vi "BSA_Setup_Options.vi"() -> (0 "IP Addresses":string[](array[string]), 1 "Channel Numbers":i32[](array[numeric]), 2 "Full BSA Strings":string[](array[string]), 3 "BSA Types":string[](array[string]), 4 "Record Length":dbl[](array[numeric])=[16.0, 32.0, 64.0, 128.0, 256.0, 512.0, 1024.0])   [LabVIEW 2022 SP3]
uses:
  <vilib>/Utility/error.llb/Trim Whitespace One-Sided.vi
  Globals/Constants_global.vi
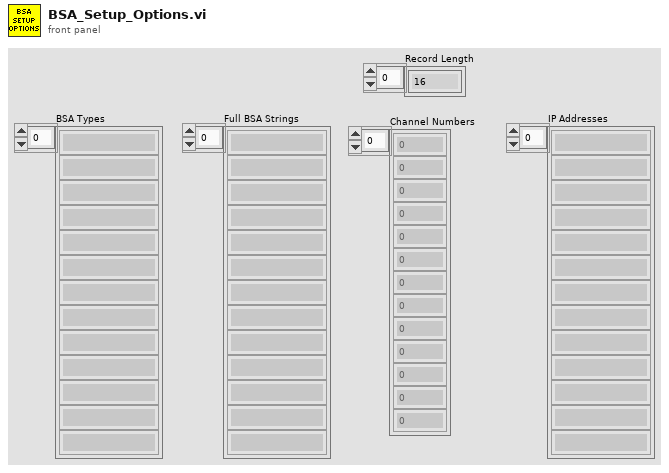
[diagram p1: front panel]
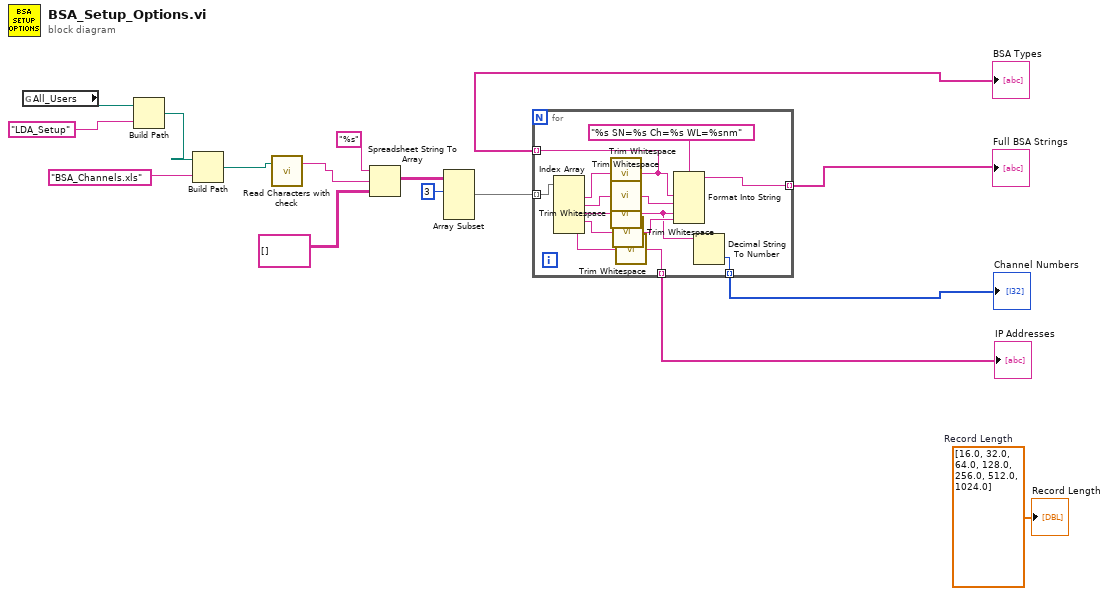
[diagram p0: block diagram]
diagram:
  w12 = dbl[] [16.0, 32.0, 64.0, 128.0, 256.0, 512.0, 1024.0]  # Record Length
  n1 = global read "Constants_global.vi" "All_Users"() -> (w11:path)
  n2 = Build Path(base path=w11, name or relative path="LDA_Setup") -> (appended path=w10:path)
  n3 = Build Path(base path=w10, name or relative path="BSA_Channels.xls") -> (appended path=w2:path)
  n4 = call "Read Characters with check.vi"("file (use dialog)"=w2) -> ("Read String"=w1:string)  [unwired: 1 in, 1 out]
  n5 = Spreadsheet String To Array(format string="%s", spreadsheet string=w1, array type (2D Dbl)=string[][] []) -> (array=w6:string[][])  [unwired: 1 in]
  n6 = Array Subset(array=w6, index (row)=3 ("index")) -> (w8:string[][])  [unwired: 3 in]
  n7 = for {
    tunnel: w8 -> [w30] mode=indexing
    tunnel: [w28] -> w16 mode=indexing
    tunnel: [w19] -> w14 mode=indexing
    tunnel: [w21] -> w15 mode=indexing
    tunnel: [w17] -> w13 mode=indexing
    n8 = Index Array(array=w30) -> (element #1=w22:string, element #2=w27:string, element #3=w25:string, element #4=w24:string, element #5=w20:string)  [unwired: 5 in]
    n9 = call <vilib>:"Trim Whitespace.vi"("string"=w22) -> ("trimmed string"=w21:string)  [unwired: 1 in]
    n10 = call <vilib>:"Trim Whitespace.vi"("string"=w27) -> ("trimmed string"=w26:string)  [unwired: 1 in]
    n11 = call <vilib>:"Trim Whitespace.vi"("string"=w25) -> ("trimmed string"=w18:string)  [unwired: 1 in]
    n12 = call <vilib>:"Trim Whitespace.vi"("string"=w24) -> ("trimmed string"=w23:string)  [unwired: 1 in]
    n13 = call <vilib>:"Trim Whitespace.vi"("string"=w20) -> ("trimmed string"=w19:string)  [unwired: 1 in]
    n14 = Format Into String(format string="%s SN=%s Ch=%s WL=%snm", w21, w26, w18, w23) -> (resulting string=w28:string)  [unwired: 2 in, 1 out]
    n15 = Decimal String To Number(string=w18) -> (number=w17:i32)  [unwired: 2 in, 1 out]
  }
  "Channel Numbers" <- w13
  "BSA Types" <- w15
  "IP Addresses" <- w14
  "Full BSA Strings" <- w16
  "Record Length" <- w12
